vi "saveAsEvent.vi"(8 "error in (no error)":errorcluster, 11 "WinX32Settings in":refnum<class "WinX32Settings.lvclass">) -> (0 "error out":errorcluster, 3 "WinX32Settings out":refnum<class "WinX32Settings.lvclass">)   [LabVIEW 2011, in "Tools.lvlib" / "Settings.lvlib" / "WinX32Settings.lvclass"]
uses:
  WinX32Settings.lvclass
  WinX32Settings.lvclass/WinX32Settings.ctl
  SettingsViewer/settingsViewer.lvclass
  Filing.lvlib
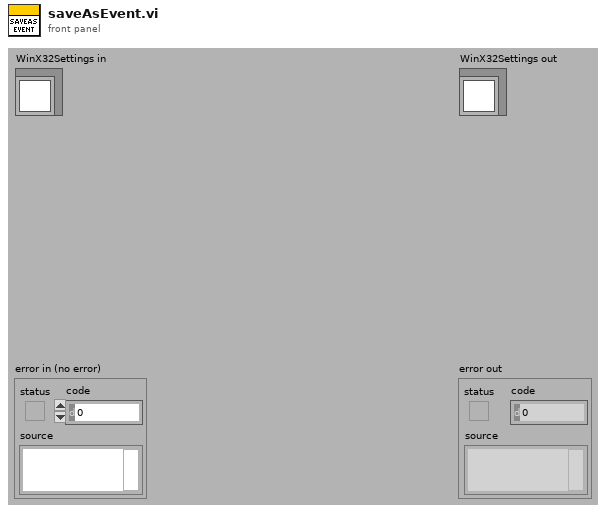
[diagram p1: front panel]
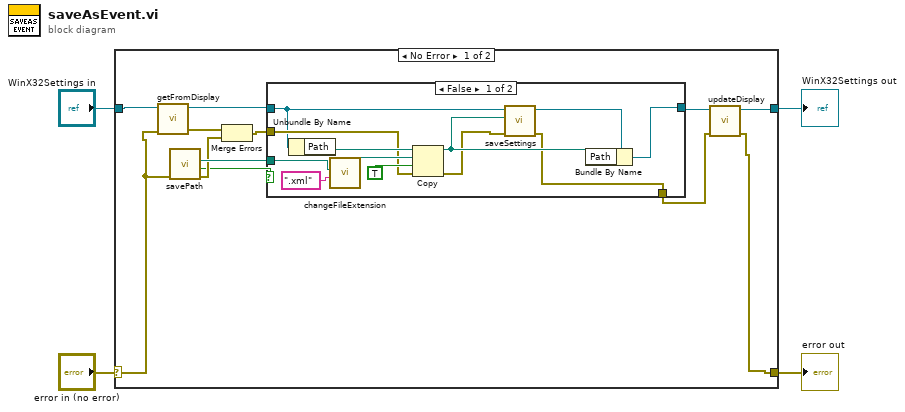
[diagram p0: block diagram]
diagram:
  n1 = case shown="No Error" "error in (no error)" {
    selector: "error in (no error)" -> [w7 w32]
    tunnel: [w10 w32] -> w2
    tunnel: [w11 w31] -> w1
    tunnel: "WinX32Settings in" -> [w8 w31]
    frame No Error {
      n2 = call "getFromDisplay.vi"("error in (no error)"=w7, "WinX32Settings in"=w8) -> ("error out"=w6:errorcluster, "WinX32Settings out"=w5:refnum<class "WinX32Settings.lvclass">)  [unwired: 8 in]
      n3 = call "savePath.vi"("error in (no error)"=w7) -> ("error out"=w15:errorcluster, "cancelled"=w14:bool, "Path out"=w16:path)  [unwired: 8 in]
      n4 = Merge Errors(w6, w15) -> (w13:errorcluster)
      n5 = case shown="False" w14 {
        tunnel: [w18 w29] -> w9
        tunnel: w5 -> [w17 w30]
        tunnel: [w28 w30] -> w12
        tunnel: w16 -> [w26 _]
        tunnel: w13 -> [w22 w29]
        frame False {
          n6 = Unbundle By Name(w17) -> ("Path"=w25:path)
          n7 = call "changeFileExtension.vi"("extension"=".xml", "Path"=w26) -> ("Path out"=w24:path)  [unwired: 9 in]
          n8 = Copy(8:w22, 9:TRUE, 10:w24, 11:w25) -> (0:w19:errorcluster, 3:w20:path)  [unwired: 1 in, 1 out]
          n9 = call-dynamic "saveSettings.vi"("error in (no error)"=w19, "Path"=w20, "WinX32Settings in"=w17) -> ("error out"=w18:errorcluster, "WinX32Settings out"=w21:refnum<class "WinX32Settings.lvclass">)  [unwired: 7 in]
          n10 = Bundle By Name(cluster=w21, "Path"=w20) -> (w28:refnum<class "WinX32Settings.lvclass">)
        }
        frame True {
        }
      }
      n11 = call "updateDisplay.vi"("error in (no error)"=w9, "WinX32Settings in"=w12) -> ("error out"=w10:errorcluster, "WinX32Settings out"=w11:refnum<class "WinX32Settings.lvclass">)  [unwired: 8 in]
    }
    frame Error {
    }
  }
  "error out" <- w2
  "WinX32Settings out" <- w1
